vi "Calculate Next Distance & Bearing.vi"(8 "Current Longitude":dbl, 9 "Destination Longitude":dbl, 10 "Current Latitude":dbl, 11 "Destination Latitude":dbl format="%#_11g") -> (3 "Distance to Next Destination (km)":dbl format="%#_21g", 5 "delLong":dbl, 7 "delLat":dbl)   [LabVIEW 2011]
uses:
  <vilib>/express/express arith-compare/Formula/XNode/ExpressFormulaBlockNode.xnode
panel:
  out "Result":dbl format="%#_23g"
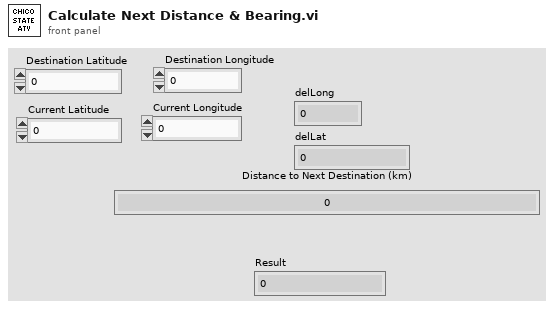
[diagram p1: front panel]
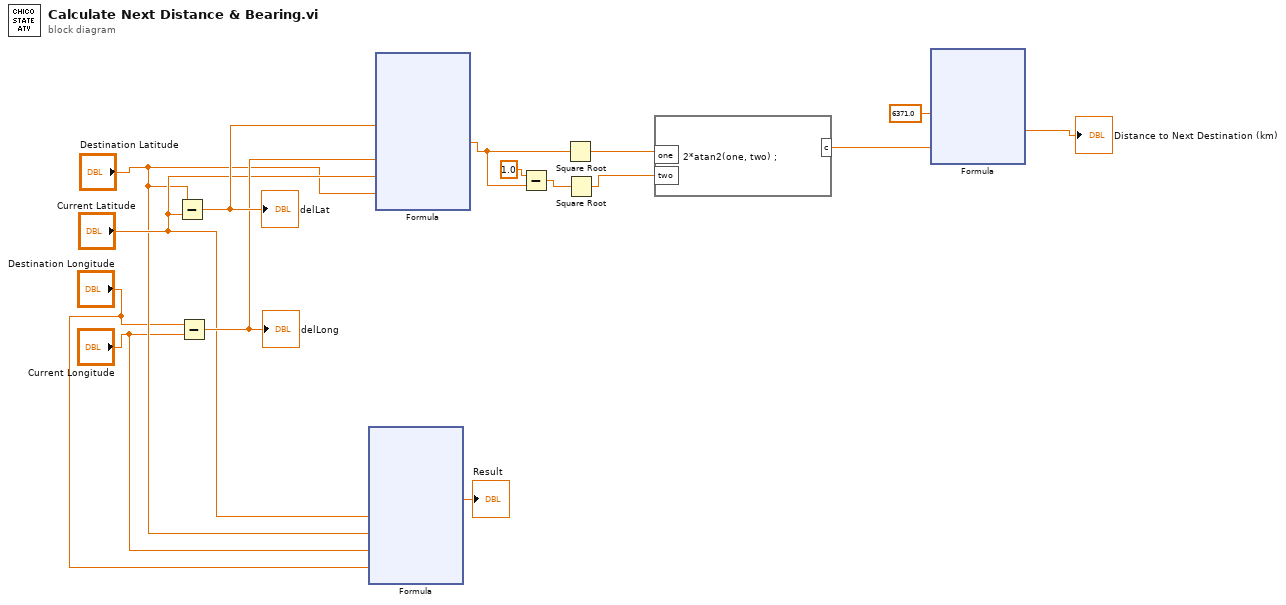
[diagram p0: block diagram]
diagram:
  n1 = Subtract(x="Destination Latitude", y="Current Latitude") -> (x-y=w7:dbl)
  "delLat" <- w7
  n2 = Subtract(x="Destination Longitude", y="Current Longitude") -> (x-y=w6:dbl)
  "delLong" <- w6
  n3 = xnode "Formula"("Lat1"="Current Latitude", "Lat2"="Destination Latitude", "Lon1"="Current Longitude", "Lon2"="Destination Longitude") -> ("Result"=→"Result":dbl)  [unwired: 1 in, 1 out]
  n4 = xnode "Formula"("delLat"=w7, "delLong"=w6, "lat1"="Current Latitude", "lat2"="Destination Latitude") -> ("Result"=w9:dbl)  [unwired: 1 in, 1 out]
  n5 = Subtract(x=1.0, y=w9) -> (x-y=w8:dbl)
  n6 = Square Root(x=w9) -> (sqrt(x)=w11:dbl)
  n7 = Square Root(x=w8) -> (sqrt(x)=w12:dbl)
  n8 = formula code="c = 2*atan2(one, two) ;"("one"=w11, "two"=w12) -> ("c"=w14:dbl)
  n9 = xnode "Formula"("R"=6371.0, "c"=w14) -> ("Result"=→"Distance to Next Destination (km)":dbl)  [unwired: 1 in, 1 out]
